vi "Get RGB.vi"(0 "comm interface in":refnum<class "Pixy Com.lvclass">, 5 "x":u16 max=315, 7 "y":u16 max=207, 9 "saturate?":bool, 11 "error in":errorcluster) -> (4 "comm interface out":refnum<class "Pixy Com.lvclass">, 6 "blue":u8, 8 "green":u8, 10 "red":u8, 15 "error out":errorcluster)   [LabVIEW 2018, in "Pixy2.lvlib"]
doc: "Gets the color (RGB) of the location specified by x, y."
uses:
  Pixy2.lvlib
  Interface/Pixy Com.lvclass
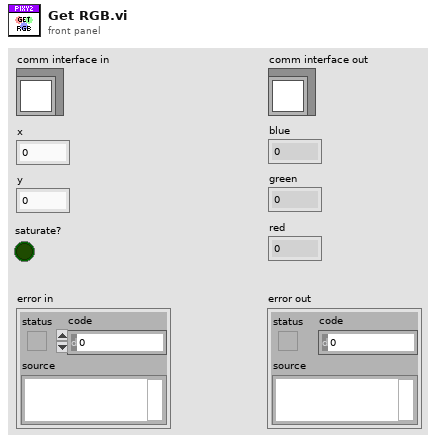
[diagram p1: front panel]
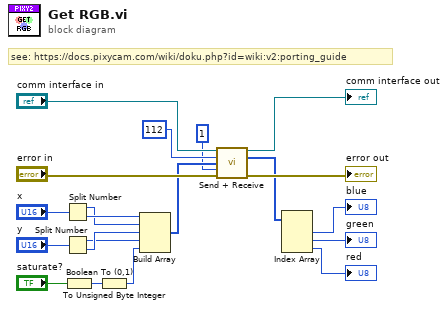
[diagram p0: block diagram]
diagram:
  # "see: https://docs.pixycam.com/wiki/doku.php?id=wiki:v2:porting_guide"
  n1 = Split Number(x="x") -> (hi(x)=w19:u8, lo(x)=w20:u8)
  n2 = Split Number(x="y") -> (hi(x)=w17:u8, lo(x)=w18:u8)
  n3 = Boolean To (0,1)(Boolean="saturate?") -> (0, 1=w13:i16)
  n4 = To Unsigned Byte Integer(number=w13) -> (unsigned 8bit integer=w12:u8)
  n5 = Build Array(w20, w19, w18, w17, w12) -> (w4:u8[])
  n6 = call "Send + Receive.vi"("comm interface in"="comm interface in", "type"=u8 112, "payload"=w4, "expected response"=u8 1 ("expected type"), "error in"="error in") -> ("comm interface out"=→"comm interface out":refnum<class "Pixy Com.lvclass">, "received"=w1:u8[], "error out"=→"error out":errorcluster)  [unwired: 8 in]
  n7 = Index Array(array=w1) -> (element #1=→"blue":u8, element #2=→"green":u8, element #3=→"red":u8)  [unwired: 3 in]
